vi "TestGetFanControlStatus.vi"() -> ()   [LabVIEW 2012]
panel:
  out "Fan Control Status   2":T1 {"Reserved" format="%0d"; "FanActual" format="%0d"; "FanSetPoint" format="%0d"; "FanStep" format="%0d"; "FanMax" format="%0d"; "FanMin" format="%0d"}
  out "Set Point Out":u16=48
  in  "Fan Set Point":u16=48 format="%0d"
  in  "Control mode":bool
  out "Fan Control Status":T1 {"Reserved" format="%0d"; "FanActual" format="%0d"; "FanSetPoint" format="%0d"; "FanStep" format="%0d"; "FanMax" format="%0d"; "FanMin" format="%0d"}
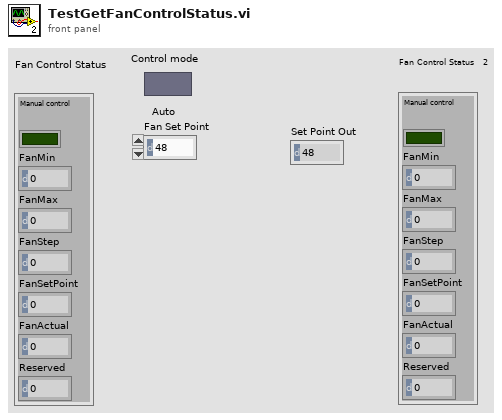
[diagram p1: front panel]
types:
  T1 = cluster{"Manual control":bool, "FanMin":u16, "FanMax":u16, "FanStep":u16, "FanSetPoint":u16, "FanActual":u16, "Reserved":u16}
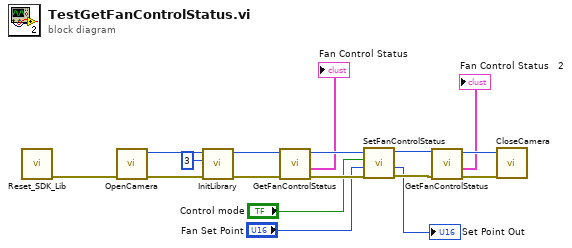
[diagram p0: block diagram]
diagram:
  n1 = call "Reset_SDK_Lib.vi"() -> ("ErrorOut"=w17:errorcluster)  [unwired: 11 in]
  n2 = call "OpenCamera.vi"("ErrorIn"=w17) -> ("ErrorOut"=w15:errorcluster, "Handle out"=w16:u64)  [unwired: 3 in, 2 out]
  n3 = call "InitLibrary.vi"("error in (no error)"=w15, "InterfaceType"=u32 3, "ph"=w16) -> ("error out"=w13:errorcluster, "hout"=w12:u64)  [unwired: 7 in]
  n4 = call "GetFanControlStatus.vi"("error in (no error)"=w13, "HandleIn"=w12) -> ("error out"=w10:errorcluster, "Fan Control Status"=→"Fan Control Status":T1, "HandleOut"=w11:u64)  [unwired: 6 in, 1 out]
  n5 = call "SetFanControlStatus.vi"("error in (no error)"=w10, "Fan Set Point"="Fan Set Point", "Control mode"="Control mode", "HandleIn"=w11) -> ("error out"=w8:errorcluster, "Set Point Out"=→"Set Point Out":u16, "HandleOut"=w9:u64)  [unwired: 4 in, 1 out]
  n6 = call "GetFanControlStatus.vi"("error in (no error)"=w8, "HandleIn"=w9) -> ("error out"=w6:errorcluster, "Fan Control Status"=→"Fan Control Status   2":T1, "HandleOut"=w7:u64)  [unwired: 6 in, 1 out]
  n7 = call "CloseCamera.vi"("ErrorIn"=w6, "Handle in"=w7) -> ()  [unwired: 1 in, 3 out]
